vi "DELETE.vi"(6 "timeout (10000)":i32=10000, 7 "output file":path=path "", 8 "error in (no error)":errorcluster, 10 "url":string, 11 "HTTP Client Base in":refnum<class "LabVIEW HTTP Client.lvclass">) -> (0 "error out":errorcluster, 1 "body":string, 2 "headers":string, 3 "HTTP Client Base out":refnum<class "LabVIEW HTTP Client.lvclass">, 4 "status code":u32)   [LabVIEW 2020, in "HTTP Client Abstract.lvlib" / "LabVIEW HTTP Client.lvclass"]
uses:
  LabVIEW HTTP Client.lvclass
  LabVIEW HTTP Client.lvclass/LabVIEW HTTP Client.ctl
  <vilib>/httpClient/LabVIEWHTTPClient.lvlib
  Abstract HTTP Client/Abstract HTTP Client.lvclass
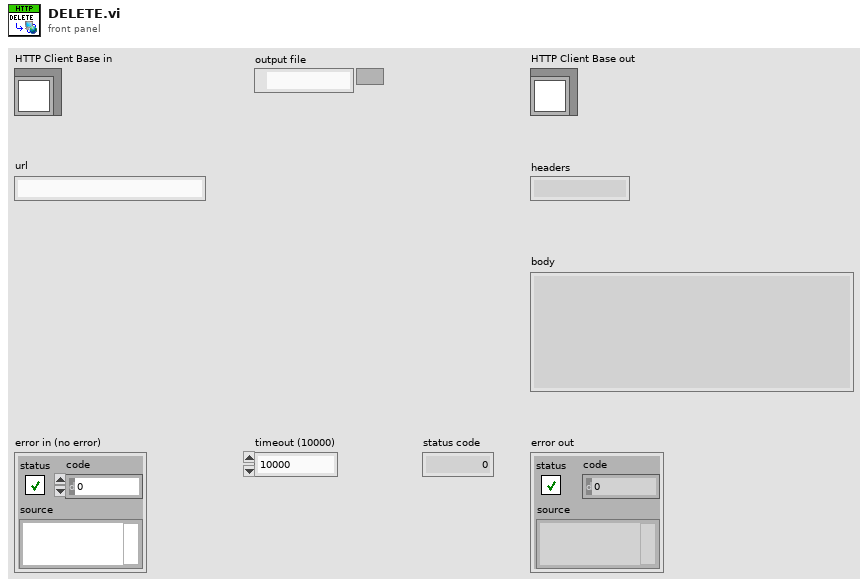
[diagram p1: front panel]
types:
  T1 = typedef "LabVIEWHTTPClient.lvlib/ClientHandle.ctl" = refnum<k1>
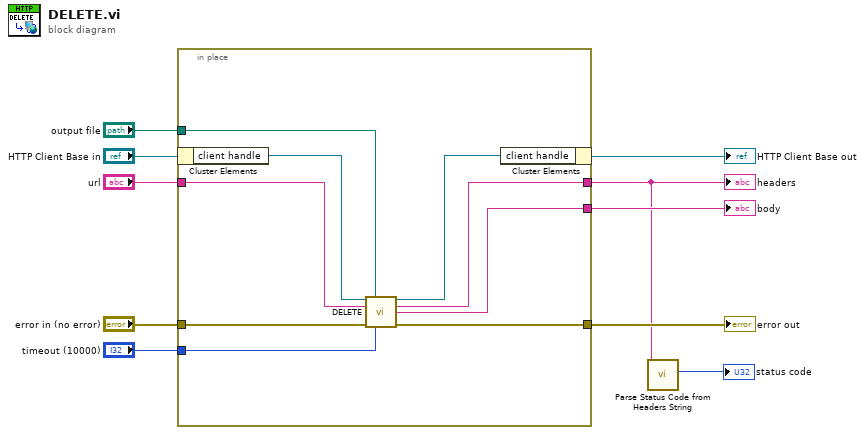
[diagram p0: block diagram]
diagram:
  n1 = in-place {
    in-place-border: "error in (no error)" -> [w19]
    in-place-border: [w18] -> w8
    in-place-border: "output file" -> [w15]
    in-place-border: "url" -> [w14]
    in-place-border: "timeout (10000)" -> [w13]
    in-place-border: [w12] -> w1
    in-place-border: [w11] -> w3
    n2 = in-place-cluster #1("HTTP Client Base in") -> ("client handle"=w17:T1)
    n3 = call <vilib>:"DELETE.vi"("client handle"=w17, "output file"=w15, "url"=w14, "error in (no error)"=w19, "timeout (10000)"=w13) -> ("client handle out"=w16:T1, "headers"=w12:string, "body"=w11:string, "error out"=w18:errorcluster)  [unwired: 7 in]
    n4 = in-place-cluster #1("client handle"=w16) -> (→"HTTP Client Base out":refnum<class "LabVIEW HTTP Client.lvclass">)
  }
  "error out" <- w8
  "headers" <- w1
  "body" <- w3
  n5 = call "Parse Status Code from Headers String.vi"("headers in"=w1) -> ("status code"=→"status code":u32)  [unwired: 10 in]
